vi "attribute_read_int32_simple.vi"(5 "Repeated Capability":string, 7 "Attribute":T1={"Identifier"="", "Descriptive name"="", "Data Type"=enum."Integer 32", "Command"="", "Access"=2, "Range Table"="", "Read Callback"="", "Write Callback"="", "Range Callback"="", "Check Callback"="", "Rngtable Callback"="", "Coerce Callback"="", "Supported Models"="", "Instrument Options"="", "Repeated Capabilities"="", "Check Status Callback"="", "Index"=0, "Flag: OPC Wait"=FALSE, "Flag: Dont check status"=FALSE, "Flag: Cache Only"=FALSE} {"Access" items=["Read Only", "Write Only", "Read/Write"]}, 8 "error in":errorcluster, 10 "Direct Attribute ID (\"\")":string, 11 "VISA resource name":refnum<visa-resource-name>) -> (0 "error out":errorcluster, 2 "int32 out":i32, 3 "VISA resource name out":refnum<visa-resource-name>)   [LabVIEW 2014, in "rszvl_rsidr_core.lvlib"]
uses:
  rszvl_rsidr_core.lvlib
  type_Attribute.ctl
  type_Attribute_Data_Type.ctl
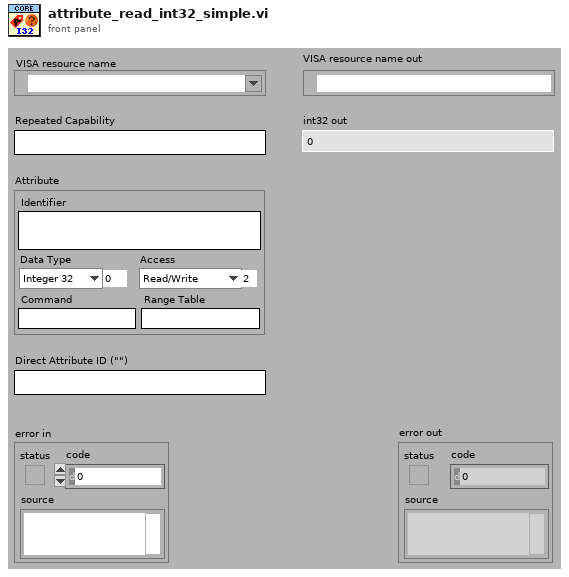
[diagram p1: front panel]
types:
  T1 = typedef "rszvl_rsidr_core.lvlib/type_Attribute.ctl" = cluster{"Identifier":string, "Descriptive name":string, "Data Type":T2, "Command":string, "Access":u16, "Range Table":string, "Read Callback":string, "Write Callback":string, "Range Callback":string, "Check Callback":string, "Rngtable Callback":string, "Coerce Callback":string, "Supported Models":string, "Instrument Options":string, "Repeated Capabilities":string, "Check Status Callback":string, "Index":i32, "Flag: OPC Wait":bool, "Flag: Dont check status":bool, "Flag: Cache Only":bool}
  T2 = typedef "rszvl_rsidr_core.lvlib/type_Attribute_Data_Type.ctl" = enum16{"Integer 32", "Double", "String", "Boolean", "None", "Integer 64"}
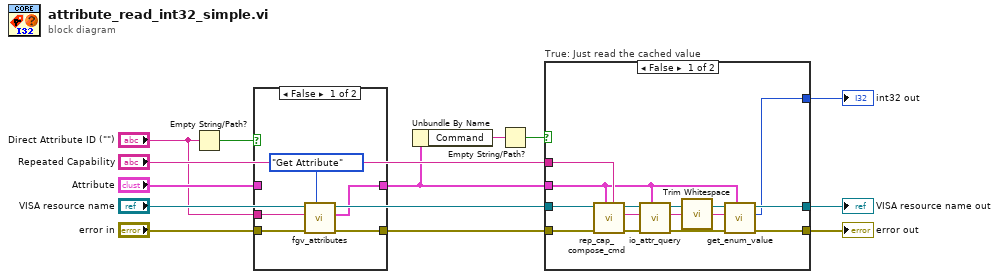
[diagram p0: block diagram]
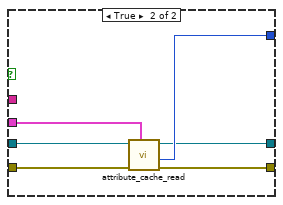
[diagram p3: hidden frame]
diagram:
  n1 = Empty String/Path?(string/path="Direct Attribute ID (\"\")") -> (empty?=w6:bool)
  n2 = case shown="False" w6 {
    tunnel: "error in" -> [w18 w19]
    tunnel: [w17 w19] -> w10
    tunnel: "Direct Attribute ID (\"\")" -> [w16 _]
    tunnel: "Attribute" -> [_ w20]
    tunnel: [w14 w20] -> w5
    frame False {
      n3 = call "fgv_attributes.vi"("Operation"=enum16{"Initialize", "Get Attribute"}."Get Attribute", "error in"=w18, "Attribute ID in"=w16) -> ("error out"=w17:errorcluster, "Attribute out"=w14:T1)  [unwired: 6 in, 1 out]
    }
    frame True {
    }
  }
  n4 = Unbundle By Name(w5) -> ("Command"=w4:string)
  n5 = Empty String/Path?(string/path=w4) -> (empty?=w3:bool)
  n6 = case "True: Just read the cached value" shown="False" w3 {
    tunnel: "Repeated Capability" -> [w34 _]
    tunnel: [w33 w36] -> w2
    tunnel: [w32 w35] -> w1
    tunnel: [w31 w37] -> w12
    tunnel: "VISA resource name" -> [w30 w39]
    tunnel: w10 -> [w29 w40]
    tunnel: w5 -> [w28 w38]
    frame False {
      n7 = call "rep_cap_compose_cmd.vi"("Repeated Capability"=w34, "Attribute"=w28, "error in"=w29, "VISA resource name"=w30) -> ("error out"=w27:errorcluster, "Command out"=w26:string, "VISA resource name out"=w25:refnum<visa-resource-name>)  [unwired: 5 in]
      n8 = call "io_attr_query.vi"("Attribute"=w28, "error in"=w27, "write buffer"=w26, "VISA resource name"=w25) -> ("error out"=w24:errorcluster, "read buffer"=w22:string, "VISA resource name out"=w23:refnum<visa-resource-name>)  [unwired: 5 in]
      n9 = call "Trim Whitespace.vi"("string"=w22) -> ("trimmed string"=w21:string)  [unwired: 1 in]
      n10 = call "get_enum_value.vi"("Attribute"=w28, "error in"=w24, "String Value"=w21, "VISA resource name"=w23) -> ("error out"=w33:errorcluster, "I32 output"=w31:i32, "VISA resource name out"=w32:refnum<visa-resource-name>)  [unwired: 5 in]
    }
    frame True {
      n11 = call "attribute_cache_read.vi"("Attribute"=w38, "error in"=w40, "VISA resource name"=w39) -> ("error out"=w36:errorcluster, "Integer 32 out"=w37:i32, "VISA resource name out"=w35:refnum<visa-resource-name>)  [unwired: 1 in, 5 out]
    }
  }
  "error out" <- w2
  "VISA resource name out" <- w1
  "int32 out" <- w12
